vi "Multi_analog_acquire.vi"() -> ()   [LabVIEW 2012]
uses:
  <vilib>/Utility/file.llb/Write To Spreadsheet File (DBL).vi
  <vilib>/MakerHub/LINX/Public/Peripherals/Analog/Analog Read N Chans.vi
  <vilib>/MakerHub/LINX/LMH-LINX.lvlib
panel:
  in  "Acquisition Interval":u32=50 min=50 max=10000 step=50 format="%.0fms"
  out "Status":bool caption="Connected?"
  in  "Save As":bool
  in  "Exit":bool
  out "Acquire \nPlot":T1(graph)
  in  "Acquire":bool
  in  "Serial Port":refnum<visa-resource-name>="N/A"
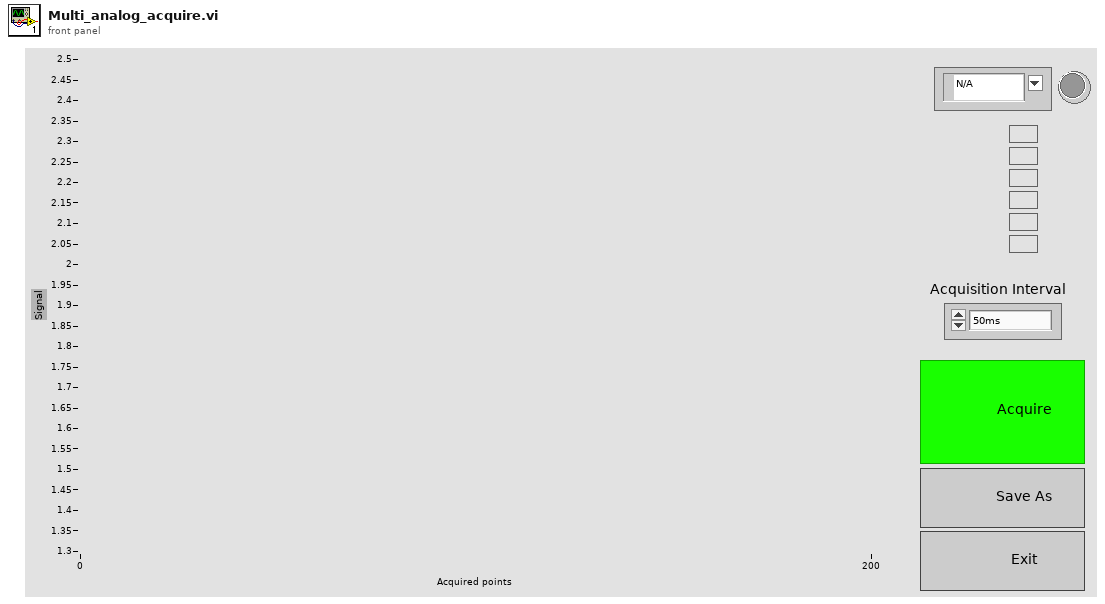
[diagram p1: front panel]
types:
  T1 = cluster{"Numeric Control":dbl, "Numeric Control":dbl, "Numeric Control":dbl, "Numeric Control":dbl, "Numeric Control":dbl, "Numeric Control":dbl}
  T2 = typedef "LMH-LINX.lvlib/LINX Ref.ctl" = cluster{"Platform":T3, "Interface":T4, "LINX Device Config":T5}
  T3 = typedef "LMH-LINX.lvlib/Platform.ctl" = enum16{"LINX", "myRIO"}
  T4 = typedef "LMH-LINX.lvlib/Interface.ctl" = enum16{"Serial", "TCP"}
  T5 = typedef "LMH-LINX.lvlib/Device.lvlib/LINX Device Config.ctl" = cluster{"Interface":T4, "COM Port":refnum<visa-resource-name>, "TCP Configuration":T6, "Device Family":u8, "Device ID":u8, "Device Name":string, "TCP Ref":refnum<k5>, "Channels":T7}
  T6 = typedef "LMH-LINX.lvlib/Device.lvlib/TCP Config.ctl" = cluster{"IP Address":string, "Port":u16}
  T7 = typedef "LMH-LINX.lvlib/Channels.ctl" = cluster{"DI":u8[], "DO":u8[], "AI":u8[], "AO":u8[], "PWM":u8[], "QE":u8[], "UART":u8[], "I2C 2":u8[], "SPI":u8[], "CAN":u8[], "Servo":u8[], "AI Ref (V)":dbl, "AO Ref (V)":dbl, "AO Resolution (Bits)":u8}
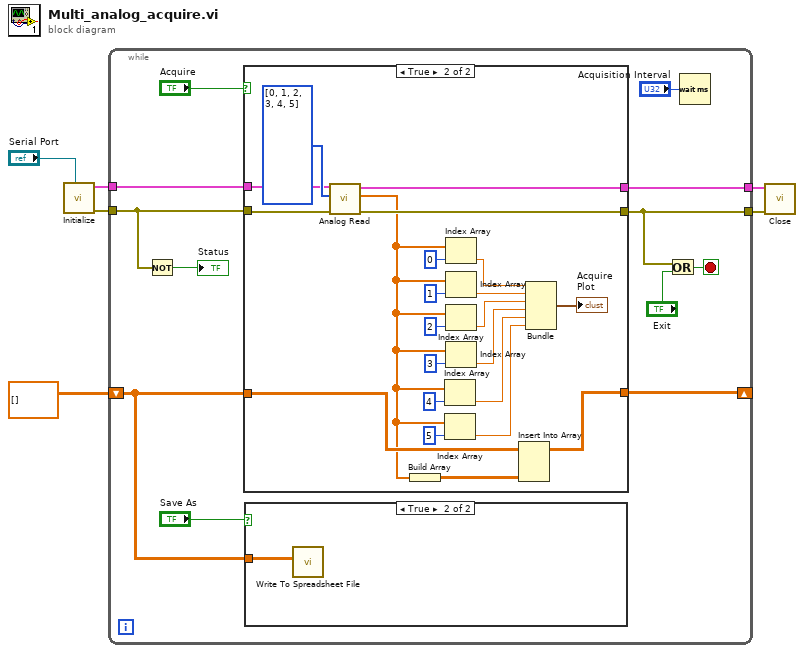
[diagram p0: block diagram]
diagram:
  n1 = call <vilib>:"Initialize.vi"("Serial Port"="Serial Port") -> ("Error Out"=w4:errorcluster, "LINX Ref"=w5:T2)  [unwired: 8 in, 1 out]
  n2 = while {
    tunnel: w5 -> [w17]
    tunnel: w4 -> [w11]
    tunnel: [w16] -> w1
    tunnel: [w13] -> w2
    shift-right: [w9] -> _
    shift-left: dbl[][] [] -> [w8]
    stop <- w14 stop-if-true
    n3 = Not(x=w11) -> (.not. x?=→"Status":bool)
    n4 = case shown="True" "Acquire" {
      tunnel: w17 -> [w20 w28]
      tunnel: w11 -> [w22 w30]
      tunnel: [w20 w32] -> w16
      tunnel: [w22 w31] -> w13
      tunnel: w8 -> [w21 w35]
      tunnel: [w21 w34] -> w9
      frame False {
      }
      frame True {
        n5 = call-poly <vilib>:"Analog Read.vi"("Error In"=w30, "AI Channel(s)"=u8[] [0, 1, 2, 3, 4, 5], "LINX Resource"=w28) -> ("Error Out"=w31:errorcluster, "Voltages"=w25:dbl[], "LINX Resource"=w32:T2)  [unwired: 5 in, 1 out]
        n6 = Build Array(w25) -> (w33:dbl[][])
        n7 = Index Array(array=w25, index=4) -> (element=w24:dbl)
        n8 = Index Array(array=w25, index=5) -> (element=w23:dbl)
        n9 = Index Array(array=w25, index=0) -> (element=w41:dbl)
        n10 = Index Array(array=w25, index=1) -> (element=w42:dbl)
        n11 = Index Array(array=w25, index=2) -> (element=w38:dbl)
        n12 = Index Array(array=w25, index=3) -> (element=w37:dbl)
        n13 = Insert Into Array(array=w35, new element=w33) -> (w34:dbl[][])  [unwired: 2 in]
        n14 = Bundle("Numeric Control"=w41, "Numeric Control"=w42, "Numeric Control"=w38, "Numeric Control"=w37, "Numeric Control"=w24, "Numeric Control"=w23) -> (→"Acquire \nPlot":T1)  [unwired: 1 in]
      }
    }
    n15 = case shown="True" "Save As" {
      tunnel: w8 -> [_ w19]
      frame False {
      }
      frame True {
        n16 = call-poly <vilib>:"Write To Spreadsheet File.vi"("2D data"=w19) -> ()  [unwired: 7 in, 1 out]
      }
    }
    n17 = Or(x=w13, y="Exit") -> (x .or. y?=w14:bool)
    n18 = Wait (ms)(milliseconds to wait="Acquisition Interval") -> ()  [unwired: 1 out]
  }
  n19 = call <vilib>:"Close.vi"("Error In"=w2, "LINX Resource"=w1) -> ()  [unwired: 8 in, 2 out]
